vi "ApplyPreferencesToVIs.vi"(6 "Total Iteration Progress":dbl, 7 "Project":refnum<vi>, 8 "error in (no error)":errorcluster, 11 "VIs":refnum<vi>[](array[refnum])) -> (0 "error out":errorcluster, 3 "dup VIs":refnum<vi>[](array[refnum]))   [LabVIEW 2016, in "NI_NPW_Project Copying.lvlib"]
uses:
  <resource>/dialog/NewProjectWizard/Project Copying/NI_NPW_Project Copying.lvlib
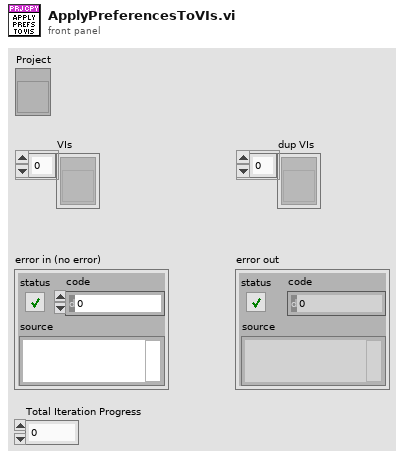
[diagram p1: front panel]
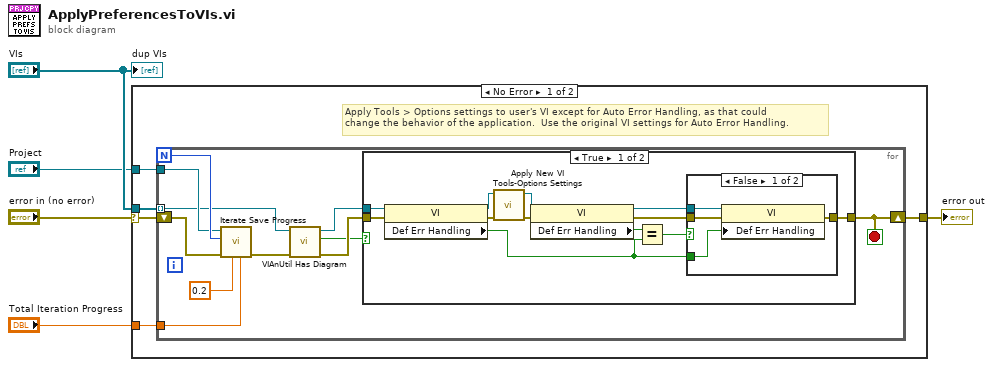
[diagram p0: block diagram]
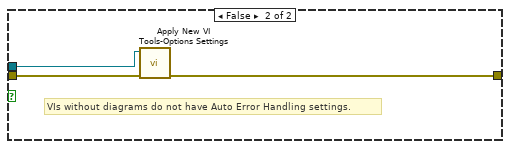
[diagram p3: hidden frame]
diagram:
  n1 = case shown="No Error" "error in (no error)" {
    selector: "error in (no error)" -> [w8 w42]
    tunnel: "VIs" -> [w10 _]
    tunnel: [w9 w42] -> w4
    tunnel: "Total Iteration Progress" -> [w7 _]
    tunnel: "Project" -> [w6 _]
    frame No Error {
      # "Apply Tools > Options settings to user's VI except for Auto Error Handling, as that could\nchange the behavior of the application.  Use the original VI settings for Auto Error Handling."
      n2 = for {
        N -> [w20]
        tunnel: w10 -> [w14] mode=indexing
        shift-right: [w19] -> w9
        shift-left: w8 -> [w21]
        tunnel: w7 -> [w18]
        tunnel: w6 -> [w16]
        stop <- w19 stop-if-true
        n3 = call <resource>:"Iterate Save Progress.vi"("Total Iteration Progress"=w18, "This Task's Percentage"=0.2, "error in (no error)"=w21, "Total Iterations (this task)"=w20, "Project"=w16) -> ("error out"=w15:errorcluster)  [unwired: 6 in]
        n4 = call <vilib>:"VIAnUtil Has Diagram.vi"("error in (no error)"=w15, "VI Ref"=w14) -> ("error out"=w13:errorcluster, "Has Diag?"=w11:bool, "dup VI Ref"=w12:refnum<vi>)  [unwired: 5 in, 2 out]
        n5 = case shown="True" w11 {
          tunnel: [w24 w41] -> w19
          tunnel: w13 -> [w23 w39]
          tunnel: w12 -> [w22 w40]
          frame True {
            n6 = property class="VI"(reference=w22, error in=w23) -> (reference out=w33:refnum<vi>, error out=w27:errorcluster, "Def Err Handling"=w28:bool)
            n7 = call <vilib>:"Apply New VI Tools-Options Settings.vi"("error in (no error)"=w27, "VI Refnum"=w33) -> ("error out"=w26:errorcluster, "dup VI Refnum"=w32:refnum<vi>)  [unwired: 8 in]
            n8 = property class="VI"(reference=w32, error in=w26) -> (reference out=w30:refnum<vi>, error out=w25:errorcluster, "Def Err Handling"=w29:bool)
            n9 = Equal?(x=w29, y=w28) -> (x = y?=w31:bool)
            n10 = case shown="False" w31 {
              tunnel: w30 -> [w37 _]
              tunnel: w28 -> [w36 _]
              tunnel: w25 -> [w35 w38]
              tunnel: [w34 w38] -> w24
              frame False {
                n11 = property class="VI"(reference=w37, error in=w35, "Def Err Handling"=w36) -> (error out=w34:errorcluster)  [unwired: 1 out]
              }
              frame True {
              }
            }
          }
          frame False {
            # "VIs without diagrams do not have Auto Error Handling settings."
            n12 = call <vilib>:"Apply New VI Tools-Options Settings.vi"("error in (no error)"=w39, "VI Refnum"=w40) -> ("error out"=w41:errorcluster)  [unwired: 8 in, 1 out]
          }
        }
      }
    }
    frame Error {
    }
  }
  "error out" <- w4
  "dup VIs" <- "VIs"
